vi "mainObjectivesRegistrationEtl.vi"() -> ()   [LabVIEW 2017]
uses:
  getComputerName.vi
  globalDevices.vi
  globalUtilities.vi
  <vilib>/Analysis/NI_AALBase.lvlib
panel:
  out "setting etl1 to":dbl
  out "folder name":string
  in  "redgreen":bool=TRUE
  out "Intensity Graph":u16[][](graph)
  out "XY Graph 6":cluster{"X":dbl, "Y":dbl}[](graph)
  out "XY Graph 5":cluster{"X":dbl, "Y":dbl}[](graph)
  out "XY Graph 4":cluster{"X":dbl, "Y":dbl}[](graph)
  out "XY Graph 3":cluster{"X":dbl, "Y":dbl}[](graph)
  out "XY Graph 2":cluster{"X":dbl, "Y":dbl}[](graph)
  out "XY Graph":cluster{"X":dbl, "Y":dbl}[](graph)
  out "curr etl0 pos (index)":i32
  out "dpt0[dpt1]":dbl[](array[numeric])=[-1.3290463804486958, -1.2316305979268645, -1.1212630461318092, -1.0138414017259925, -0.9077086052642437, -0.7879824961067727, -0.6552620830414349, -0.5431711241489464, -0.4247559983519593, -0.3094500332450975, -0.18905192370600912, -0.06093037048920009, 0.06463589071459266, 0.2196498896905996, 0.3584540083954262, 0.4919160251092355, 0.6311778325996011, 0.7706641387872266, 0.9159712492967972, 1.0737300085708255, 1.2329966463874322]
  in  "etl1 Q-1":i32=20
  out "N^2 +M galvo":i32
  out "curr. etl1 pos (index)":i32
  out "curr. galvo pos (index)":i32
  out "opendisplayvolume":bool=TRUE
  in  "frames per second":dbl=2.0
  in  "etl0 P-1":i32=40
  in  "galvo N-1":i32=3
  # "REGISTRATION BETWEEN GALVO AND CAMERA"
  # "To produce the Red-Green transformation, after running this VI with redgreen=true, use subvi/subvi-gmmreg/gmmregRegisterRedAndGreen."
  # "Acquisition parameters"
  # "# of etl \npositions to scan"
  # "40 20 for normal operation"
  # "sqrt# of galvo positions in grid\n(without symmetry breaking)"
  # "To set the extent of the galvo scan, use globalDevices.vi."
  # "0. No iris closed after tunable lens, lenses released, laser on, camera released."
  # "1. After the ETL scan ends, the Display Volume vi will open. Select a rectangle to locate the\n    two-photon spot.\n2. After the galvo scan ends, the Display VI will open again. Select a point where you want to shine\n    light, to test the registration."
  # "Always check that the [dpt1] values are reasonable. -->\nIf not, rerun the fits and correct, using basic/test/gaussianFitTestWithData"
  # "When this button is on, open the VI (if it hasn't opened yet by itself)\nsubvi/subvi-acquisitionUtilities/acquisitionDisplayVolume.vi"
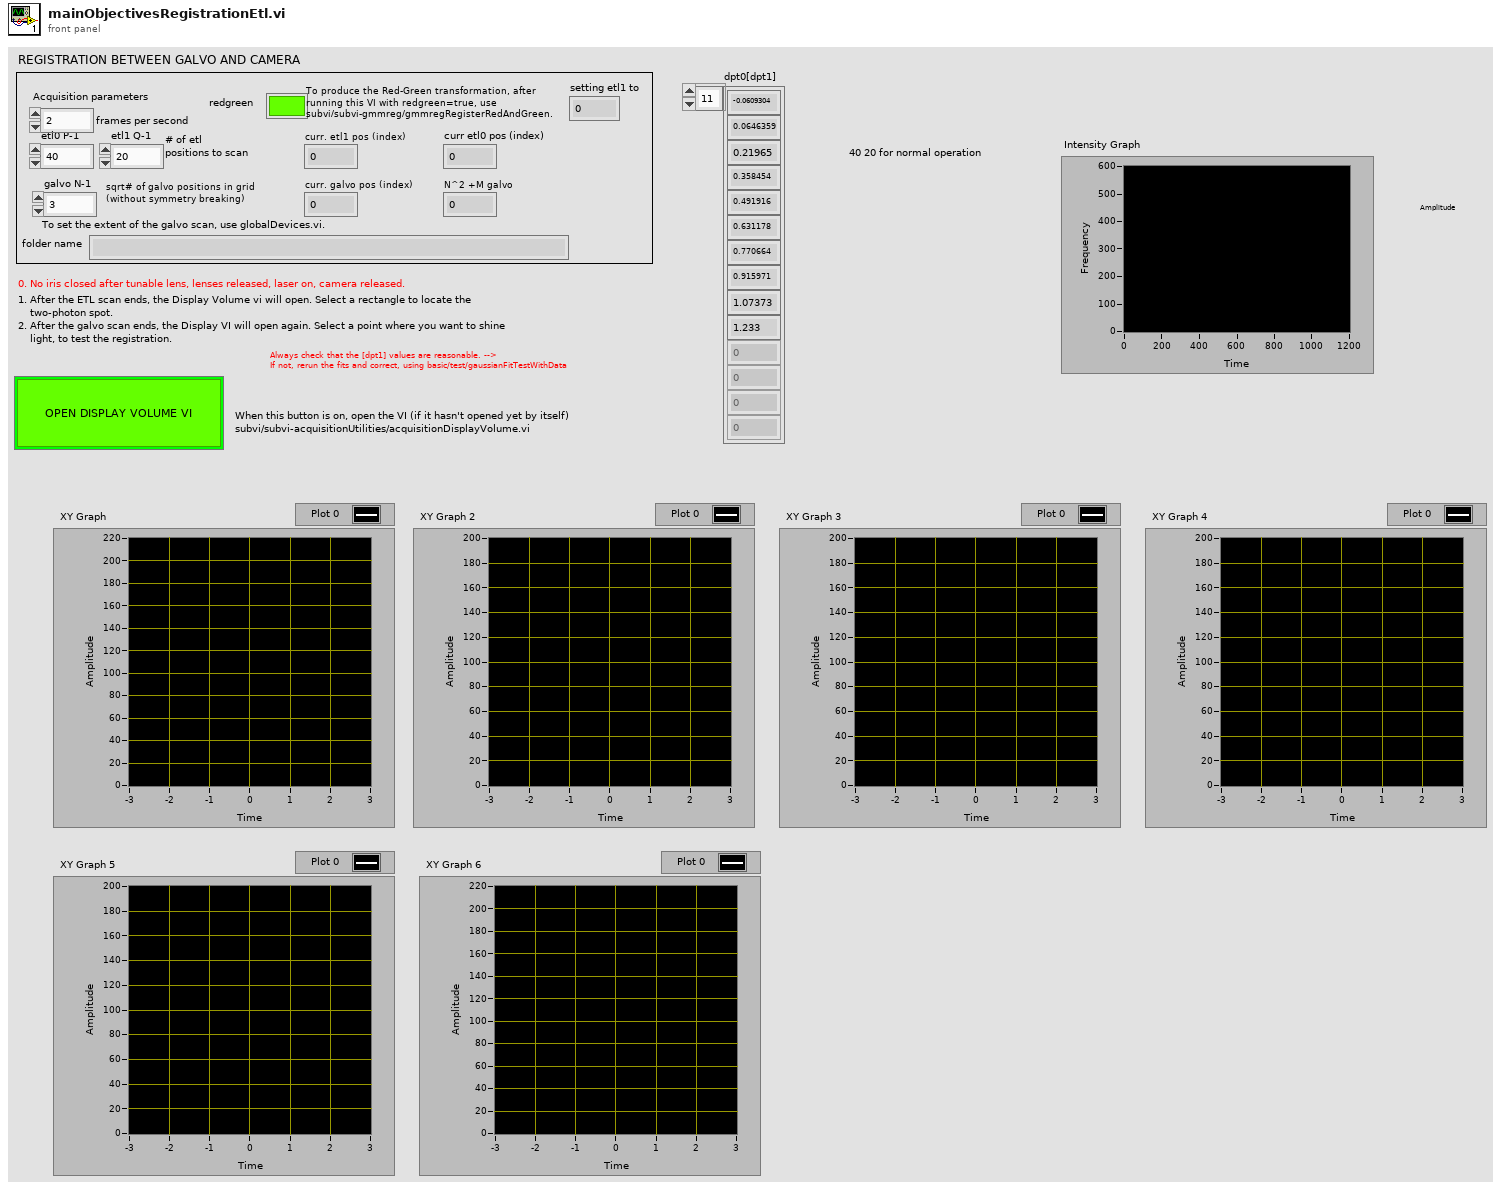
[diagram p1: front panel]
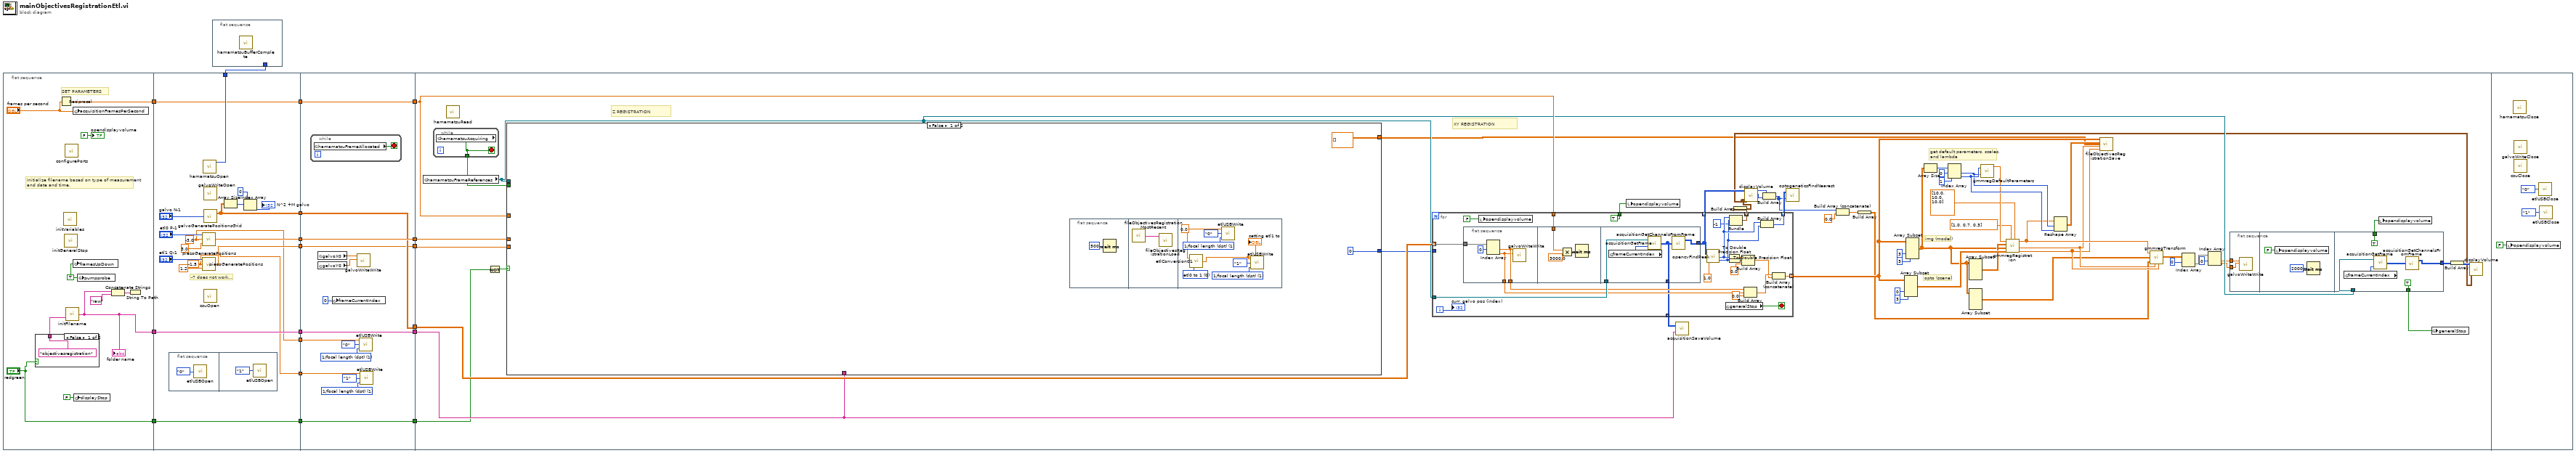
[diagram p0: block diagram]
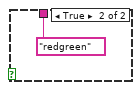
[diagram p2: hidden frame]
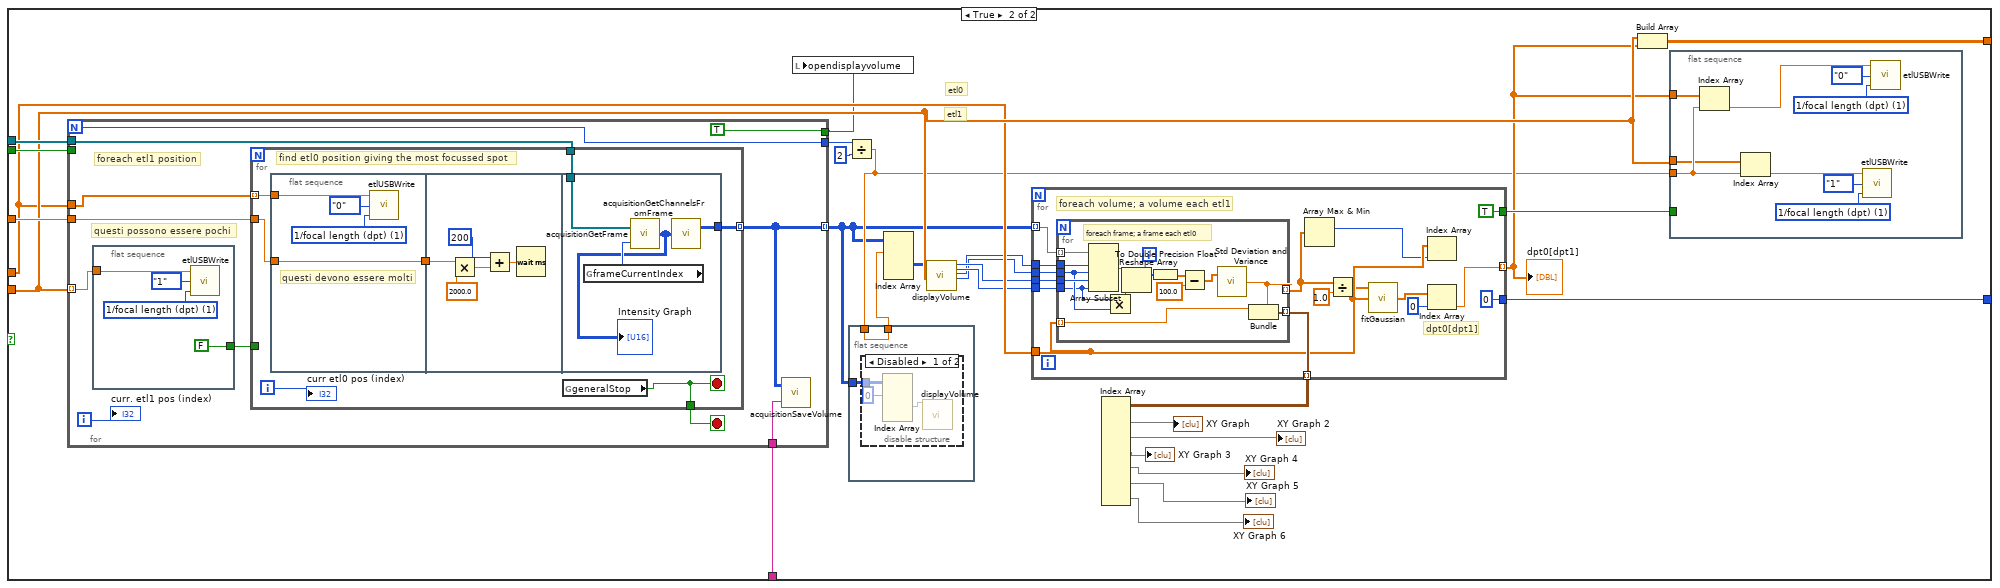
[diagram p3: hidden frame]
diagram:
  n1 = flat-sequence {
    tunnel: [w25] -> w16
    tunnel: [w22] -> w12
    tunnel: ["redgreen"] -> w7
    tunnel: [w46] -> w18
    tunnel: [w37] -> w17
    tunnel: w16 -> [w43]
    tunnel: [w43] -> w15
    tunnel: [w42] -> w14
    tunnel: [w38] -> w13
    tunnel: w12 -> [w38]
    tunnel: [w34] -> w11
    tunnel: [w32] -> w10
    tunnel: [w33] -> w9
    tunnel: [w31] -> w8
    tunnel: w7 -> [w31]
    tunnel: w17 -> [w64]
    tunnel: [w64] -> w6
    tunnel: [w63] -> w5
    tunnel: w15 -> [w63]
    tunnel: [w62] -> w4
    tunnel: w14 -> [w62]
    tunnel: [w61] -> w3
    tunnel: w13 -> [w61]
    tunnel: w11 -> [w60]
    tunnel: [w60] -> w2
    tunnel: w10 -> [w54]
    tunnel: w9 -> [w53]
    tunnel: [w50] -> w1
    tunnel: w8 -> [w50]
    tunnel: w6 -> [w69]
    tunnel: w5 -> [w117]
    tunnel: w4 -> [w119]
    tunnel: w3 -> [w68]
    tunnel: w2 -> [w70]
    tunnel: w1 -> [w67]
    frame #0 {
      w23 = TRUE ("pumpprobe")
      # "SET PARAMETERS"
      # "Initialize filename based on type of measurement\nand date and time."
      n2 = case shown="False" "redgreen" {
        tunnel: ["objectivesregistration" ("Experiment type") "redgreen" ("Experiment type")] -> w21
        frame False {
        }
        frame True {
        }
      }
      n3 = Reciprocal(x="frames per second") -> (1/x=w25:dbl)
      n4 = call "initVariables.vi"() -> ()  [unwired: 12 in]
      n5 = call "initGeneralStop.vi"() -> ()  [unwired: 1 in]
      n6 = call "configurePorts.vi"() -> ()  [unwired: 12 in]
      n7 = call "initFilename.vi"("Experiment type"=w21) -> ("folder name"=w22:string)  [unwired: 1 in]
      "folder name" <- w22
      n8 = global write "globalUtilities.vi" "framesUpDown"(w23) -> ()
      n9 = global write "globalUtilities.vi" "acquisitionFramesPerSecond"("frames per second") -> ()
      n10 = global write "globalUtilities.vi" "displayStop"(FALSE ("displayStop")) -> ()
      n11 = global write "globalUtilities.vi" "pumpprobe"(w23) -> ()
      n12 = Concatenate Strings(w22, "raw") -> (w28:string)
      n13 = String To Path(string=w28) -> ()  [unwired: 1 out]
      "opendisplayvolume" <- FALSE ("OPEN DISPLAY VOLUME")
    }
    frame #1 {
      w33 = -1.5 ("z0")
      w32 = -3.0 ("z0")
      # "-7 does not work..."
      n14 = flat-sequence {
        frame #0 {
          n15 = call "etlUSBOpen.vi"("lens"=enum16{"0", "1"}."0") -> ()  [unwired: 1 in, 1 out]
        }
        frame #1 {
          n16 = call "etlUSBOpen.vi"("lens"=enum16{"0", "1"}."1") -> ()  [unwired: 1 in, 1 out]
        }
      }
      n17 = call "piezoGeneratePositions.vi"("zf"=1.2, "z0"=w33, "M"="etl1 Q-1") -> ("positions (z)"=w34:dbl[])
      n18 = call "piezoGeneratePositions.vi"("zf"=3.0, "z0"=w32, "M"="etl0 P-1") -> ("positions (z)"=w37:dbl[])
      n19 = call "hamamatsuOpen.vi"() -> ("Handle out"=w46:u32)  [unwired: 3 out]
      n20 = call "galvoWriteOpen.vi"() -> ()  [unwired: 12 in]
      n21 = call "galvoGeneratePositionsGrid.vi"("N-1"="galvo N-1") -> ("grid"=w42:dbl[][])  [unwired: 1 out]
      n22 = call "csuOpen.vi"() -> ()  [unwired: 14 in, 2 out]
      n23 = Array Size(array=w42) -> (size(s)=w41:i32[])
      n24 = Index Array(array=w41, index=0) -> (element=→"N^2 +M galvo":i32)
    }
    frame #2 {
      w55 = u16 1 items=["position (um)", "1/focal length (dpt)"] ("mode")
      w58 = u16 1 items=["position (um)", "1/focal length (dpt)"] ("mode")
      n25 = while {
        stop <- w65 stop-if-true
        n26 = global read "globalDevices.vi" "hamamatsuFrameAllocated"() -> (w65:bool)
      }
      n27 = global read "globalDevices.vi" "galvoX0"() -> (w52:dbl)
      n28 = global read "globalDevices.vi" "galvoY0"() -> (w51:dbl)
      n29 = global write "globalUtilities.vi" "frameCurrentIndex"(0 ("frameCurrentIndex")) -> ()
      n30 = call "galvoWriteWrite.vi"("X"=w52, "Y"=w51) -> ()  [unwired: 4 in]
      n31 = call "etlUSBWrite.vi"("mode"=w55, "lens"=enum16{"0", "1"}."0", "input"=w54) -> ()  [unwired: 1 in]
      n32 = call "etlUSBWrite.vi"("mode"=w58, "lens"=enum16{"0", "1"}."1", "input"=w53) -> ()  [unwired: 1 in]
    }
    frame #3 {
      # "XY REGISTRATION"
      # "Z REGISTRATION"
      # "get default parameters, scales,\nand lambda"
      # "img (model)"
      # "opto (scene)"
      n33 = global read "globalDevices.vi" "hamamatsuFrameReferences"() -> (w96:refnum<data-value>[])
      n34 = while {
        tunnel: [w283] -> w118
        stop <- w283 stop-if-true
        n35 = global read "globalUtilities.vi" "hamamatsuAcquiring"() -> (w283:bool)
      }
      n36 = call "hamamatsuRead.vi"() -> ()  [unwired: 12 in]
      n37 = Not(x=w67) -> (.not. x?=w66:bool)
      n38 = case shown="False" w66 {
        tunnel: w118 -> [_ w158]
        tunnel: w117 -> [_ w157]
        tunnel: w96 -> [_ w156]
        tunnel: [0 w155] -> w72
        tunnel: [dbl[][] [] w154] -> w71
        tunnel: w70 -> [_ w153]
        tunnel: w69 -> [_ w150]
        tunnel: w68 -> [_ w148]
        frame False {
          n39 = flat-sequence {
            frame #0 {
              n40 = Wait (ms)(milliseconds to wait=u32 500) -> ()  [unwired: 1 out]
            }
            frame #1 {
              n41 = call "fileObjectivesRegistrationMostRecent.vi"() -> ("f"=w123:string)  [unwired: 1 in]
              n42 = call "fileObjectivesRegistrationLoad.vi"("objectiveRegistrationFilePath"=w123) -> ()  [unwired: 3 in, 6 out]
            }
            frame #2 {
              w125 = u16 0 items=["etl0 to 1", "etl1 to 0"] ("mode")
              w126 = 0.0 ("input")
              w130 = u16 1 items=["position (um)", "1/focal length (dpt)"] ("mode")
              w127 = u16 1 items=["position (um)", "1/focal length (dpt)"] ("mode")
              n43 = call "etlConversion01.vi"("mode"=w125, "in"=w126) -> ("out"=w124:dbl)
              "setting etl1 to" <- w124
              n44 = call "etlUSBWrite.vi"("mode"=w130, "lens"=enum16{"0", "1"}."0", "input"=w126) -> ()  [unwired: 1 in]
              n45 = call "etlUSBWrite.vi"("mode"=w127, "lens"=enum16{"0", "1"}."1", "input"=w124) -> ()  [unwired: 1 in]
            }
          }
        }
        frame True {
          # "etl0"
          # "etl1"
          n46 = for {
            N -> [w200]
            tunnel: w156 -> [w201]
            tunnel: w157 -> [w202]
            tunnel: [TRUE] -> w147
            tunnel: w158 -> [_]
            tunnel: [w194] -> w131 mode=indexing
            tunnel: [w200] -> w146
            tunnel: w153 -> [w199] mode=indexing
            tunnel: w150 -> [w198]
            tunnel: w148 -> [w195]
            i -> [w203]
            stop <- w196 stop-if-true
            # "foreach etl1 position"
            # "questi possono essere pochi"
            n47 = flat-sequence {
              tunnel: w199 -> [w228]
              tunnel: [FALSE] -> w197
              frame #0 {
                w226 = u16 1 items=["position (um)", "1/focal length (dpt)"] ("mode")
                n48 = call "etlUSBWrite.vi"("mode"=w226, "lens"=enum16{"0", "1"}."1", "input"=w228) -> ()  [unwired: 1 in]
              }
            }
            n49 = for {
              tunnel: w198 -> [w211] mode=indexing
              tunnel: w202 -> [w209]
              tunnel: w201 -> [w208]
              tunnel: [w207] -> w194 mode=indexing
              tunnel: w197 -> [_]
              tunnel: [w205] -> w196
              i -> [w206]
              stop <- w205 stop-if-true
              # "find etl0 position giving the most focussed spot"
              n50 = flat-sequence {
                tunnel: w211 -> [w213]
                tunnel: [w212] -> w210
                tunnel: w209 -> [w212]
                tunnel: w210 -> [w218]
                tunnel: w208 -> [w223]
                tunnel: [w222] -> w207
                frame #0 {
                  w215 = u16 1 items=["position (um)", "1/focal length (dpt)"] ("mode")
                  # "questi devono essere molti"
                  n51 = call "etlUSBWrite.vi"("mode"=w215, "lens"=enum16{"0", "1"}."0", "input"=w213) -> ()  [unwired: 1 in]
                }
                frame #1 {
                  n52 = Multiply(x=w218, y=2000.0) -> (x*y=w216:dbl)
                  n53 = Add(x=200, y=w216) -> (x+y=w220:dbl)
                  n54 = Wait (ms)(milliseconds to wait=w220) -> ()  [unwired: 1 out]
                }
                frame #2 {
                  n55 = global read "globalUtilities.vi" "frameCurrentIndex"() -> (w224:i32)
                  n56 = call "acquisitionGetFrame.vi"("index"=w224, "hamamatsuFrameReferences"=w223) -> ("frameOut"=w221:u16[][])
                  "Intensity Graph" <- w221
                  n57 = call "acquisitionGetChannelsFromFrame.vi"("frameIn"=w221) -> ("Red"=w222:u16[][])  [unwired: 1 out]
                }
              }
              n58 = global read "globalUtilities.vi" "generalStop"() -> (w205:bool)
              "curr etl0 pos (index)" <- w206
            }
            n59 = call "acquisitionSaveVolume.vi"("folder"=w195, "volume"=w194) -> ()  [unwired: 1 in]
            "curr. etl1 pos (index)" <- w203
          }
          n60 = local write "opendisplayvolume"(w147) -> ()
          n61 = Divide(x=w146, y=2) -> (x/y=w149:dbl)
          n62 = flat-sequence {
            tunnel: w149 -> [w160]
            tunnel: [w160] -> w132
            tunnel: w131 -> [w159]
            frame #0 {
              n63 = disable-structure shown="Disabled" {
                disable-tunnel: w159 -> [w163 _]
                frame Disabled {
                  n64 = Index Array(array=w163, index (dim 0)=0 ("index (vol)")) -> (element=w161:u16[][][])  [unwired: 3 in]
                  n65 = call "displayVolume.vi"("frames"=w161) -> ()  [unwired: 13 in, 6 out]
                }
                frame Enabled {
                }
              }
            }
          }
          n66 = Index Array(array=w131, index (dim 0)=w132) -> (element=w144:u16[][][])  [unwired: 3 in]
          n67 = call "displayVolume.vi"("frames"=w144, "z"=w153) -> ("X0out"=w143:i32, "deltaXout"=w142:i32, "Y0out"=w141:i32, "deltaYout"=w140:i32)  [unwired: 12 in, 2 out]
          n68 = for {
            tunnel: w131 -> [w174] mode=indexing
            tunnel: w143 -> [w179]
            tunnel: w142 -> [w178]
            tunnel: w141 -> [w177]
            tunnel: w140 -> [w176]
            tunnel: [w167] -> w151 mode=indexing
            tunnel: [0] -> w155
            tunnel: w150 -> [w169]
            tunnel: [TRUE] -> w152
            tunnel: [w170] -> w139 mode=indexing
            # "dpt0[dpt1]"
            # "foreach volume; a volume each etl1"
            n69 = for {
              tunnel: w174 -> [w193] mode=indexing
              tunnel: w179 -> [w192]
              tunnel: w178 -> [w188]
              tunnel: w177 -> [w191]
              tunnel: w176 -> [w189]
              tunnel: [w180] -> w166 mode=indexing
              tunnel: w169 -> [w186] mode=indexing
              tunnel: [w185] -> w170 mode=indexing
              # "foreach frame; a frame each etl0"
              n70 = Array Subset(array=w193, index (row)=w191, length (row)=w189, index (col)=w192, length (col)=w188) -> (w190:u16[][])
              n71 = Multiply(x=w188, y=w189) -> (x*y=w187:i32)
              n72 = Reshape Array(w190, w187) -> (w184:u16[])
              n73 = To Double Precision Float(number=w184) -> (double precision float=w183:dbl[])
              n74 = Subtract(x=w183, y=100.0) -> (x-y=w182:dbl[])
              n75 = call <vilib>:"Std Deviation and Variance.vi"("X"=w182) -> ("standard deviation"=w180:dbl)  [unwired: 1 in, 2 out]
              n76 = Bundle(w186, "standard deviation"=w180) -> (w185:cluster{dbl, "standard deviation":dbl})  [unwired: 1 in]
            }
            n77 = Array Max & Min(array=w166) -> (max index (indices)=w168:i32)  [unwired: 3 out]
            n78 = Divide(x=w166, y=1.0) -> (x/y=w165:dbl[])
            n79 = call "fitGaussian.vi"("X"=w169, "Y"=w165) -> ("x0,sigma,bg,amplitude"=w172:dbl[])  [unwired: 1 in]
            n80 = Index Array(array=w169, index=w168) -> ()  [unwired: 1 out]
            n81 = Index Array(array=w172, index=0) -> (element=w167:dbl)
          }
          "dpt0[dpt1]" <- w151
          n82 = Index Array(array=w139) -> (element #1=→"XY Graph":cluster{dbl, "standard deviation":dbl}[], element #2=→"XY Graph 2":cluster{dbl, "standard deviation":dbl}[], element #3=→"XY Graph 3":cluster{dbl, "standard deviation":dbl}[], element #4=→"XY Graph 4":cluster{dbl, "standard deviation":dbl}[], element #5=→"XY Graph 5":cluster{dbl, "standard deviation":dbl}[], element #6=→"XY Graph 6":cluster{dbl, "standard deviation":dbl}[])  [unwired: 12 in]
          n83 = Build Array(w153, w151) -> (w154:dbl[][])
          n84 = flat-sequence {
            tunnel: w151 -> [w232]
            tunnel: w149 -> [w231]
            tunnel: w153 -> [w229]
            tunnel: w152 -> [_]
            frame #0 {
              w235 = u16 1 items=["position (um)", "1/focal length (dpt)"] ("mode")
              w236 = u16 1 items=["position (um)", "1/focal length (dpt)"] ("mode")
              n85 = Index Array(array=w232, index=w231) -> (element=w230:dbl)
              n86 = Index Array(array=w229, index=w231) -> (element=w233:dbl)
              n87 = call "etlUSBWrite.vi"("mode"=w235, "lens"=enum16{"0", "1"}."1", "input"=w233) -> ()  [unwired: 1 in]
              n88 = call "etlUSBWrite.vi"("mode"=w236, "lens"=enum16{"0", "1"}."0", "input"=w230) -> ()  [unwired: 1 in]
            }
          }
        }
      }
      n89 = for {
        tunnel: w119 -> [w271] mode=indexing
        tunnel: w117 -> [w270]
        tunnel: w96 -> [w269]
        tunnel: [w266] -> w116 mode=indexing
        tunnel: [w265] -> w75 mode=indexing
        tunnel: [w257] -> w102 mode=indexing
        tunnel: [w255] -> w99 mode=indexing
        tunnel: [TRUE ("OPEN DISPLAY VOLUME")] -> w77
        tunnel: [w249] -> w73 mode=indexing
        tunnel: w72 -> [_]
        i -> [w267]
        stop <- w248 stop-if-true
        n90 = flat-sequence {
          tunnel: w271 -> [w275]
          tunnel: [w273] -> w261
          tunnel: [w272] -> w260
          tunnel: w270 -> [w277]
          tunnel: w269 -> [w281]
          tunnel: [w280] -> w266
          tunnel: [w279] -> w249
          frame #0 {
            n91 = Index Array(array=w275, index #1=0 ("index")) -> (element #1=w273:dbl, element #2=w272:dbl)  [unwired: 1 in]
            n92 = call "galvoWriteWrite.vi"("X"=w273, "Y"=w272) -> ()  [unwired: 4 in]
          }
          frame #1 {
            n93 = Multiply(x=w277, y=3000.0) -> (x*y=w276:dbl)
            n94 = Wait (ms)(milliseconds to wait=w276) -> ()  [unwired: 1 out]
          }
          frame #2 {
            n95 = global read "globalUtilities.vi" "frameCurrentIndex"() -> (w282:i32)
            n96 = call "acquisitionGetFrame.vi"("index"=w282, "hamamatsuFrameReferences"=w281) -> ("frameOut"=w279:u16[][])
            n97 = call "acquisitionGetChannelsFromFrame.vi"("frameIn"=w279) -> ("Red"=w280:u16[][])  [unwired: 1 out]
          }
        }
        n98 = local write "opendisplayvolume"(FALSE ("OPEN DISPLAY VOLUME")) -> ()
        n99 = call "opencvFindPeak.vi"("blur"=1.0, "Image (2D)"=w266) -> ("maxLocY"=w254:i32, "maxLocX"=w256:i32)
        n100 = global read "globalUtilities.vi" "generalStop"() -> (w248:bool)
        n101 = To Double Precision Float(number=w256) -> (double precision float=w263:dbl)
        n102 = To Double Precision Float(number=w254) -> (double precision float=w262:dbl)
        n103 = Bundle("maxLocX"=w256, "maxLocY"=w254, -1) -> (w265:cluster{"maxLocX":i32, "maxLocY":i32, i32})  [unwired: 1 in]
        n104 = Build Array(w263, w262, 0.0 ("element")) -> (w253:dbl[])
        n105 = Build Array(w261, w260, 0.0 ("element")) -> (w258:dbl[])
        n106 = Build Array(w256, w254) -> (w255:i32[])
        n107 = Build Array (concatenate)(w258, w253) -> (w257:dbl[])
        "curr. galvo pos (index)" <- w267
      }
      n108 = local write "opendisplayvolume"(w77) -> ()
      n109 = call "acquisitionSaveVolume.vi"("folder"=w68, "volume"=w73) -> ()  [unwired: 1 in]
      n110 = Build Array(w75) -> (w74:cluster{"maxLocX":i32, "maxLocY":i32, i32}[][])
      n111 = call "displayVolume.vi"("frames"=w116, "overlay (z:-1 all planes)"=w74) -> ("X0out"=w115:i32, "Y0out"=w114:i32)  [unwired: 12 in, 4 out]
      n112 = Build Array(w115, w114) -> (w81:i32[])
      n113 = call "optogeneticsFindNearest.vi"("point"=w81, "points"=w99) -> ()  [unwired: 1 out]
      n114 = Build Array (concatenate)(w81, 0.0) -> (w79:dbl[])
      n115 = Build Array(w79) -> (w78:dbl[][])
      n116 = Array Subset(array=w102, index (col)=0 ("index"), length (col)=3 ("length")) -> (w91:dbl[][])  [unwired: 2 in]
      n117 = Array Subset(array=w102, index (col)=3 ("index"), length (col)=3 ("length")) -> (w89:dbl[][])  [unwired: 2 in]
      n118 = Array Size(array=w89) -> (size(s)=w109:i32[])
      n119 = Index Array(array=w109, index #1=0 ("index"), index #2=1 ("index")) -> (element #1=w111:i32, element #2=w112:i32)
      n120 = Array Subset(array=w89) -> (w88:dbl[][])  [unwired: 4 in]
      n121 = Array Subset(array=w89) -> (w90:dbl[][])  [unwired: 4 in]
      n122 = call "gmmregDefaultParameters.vi"("D (3)"=w112, "nctrlPts"=w111) -> ("param0"=w110:dbl[])  [unwired: 3 out]
      n123 = call "gmmregRegistration.vi"("lambda"=dbl[] [10.0, 10.0, 10.0], "scale"=dbl[] [1.0, 0.7, 0.3], "scene"=w91, "model"=w89, "ctrlPoints"=w90, "param0"=w110) -> ("denormParams out"=w92:dbl[], "normParams out"=w100:dbl[], "param0 out"=w101:dbl[])  [unwired: 2 in, 1 out]
      n124 = Reshape Array(w101, w111, w112) -> (w113:dbl[][])
      n125 = call "fileObjectivesRegistrationSave.vi"("xyz(opto)xyz(img)"=w102, "param"=w113, "normParam"=w100, "denormParam"=w92, "z(opto)z(img)"=w71) -> ()  [unwired: 1 in]
      n126 = call "gmmregTransform.vi"("param0"=w101, "ctrlPts"=w88, "pts"=w78, "normParams"=w100, "denormParams"=w92) -> ("out"=w98:dbl[][])  [unwired: 4 in]
      n127 = Index Array(array=w98, index (row)=0) -> (element=w87:dbl[])  [unwired: 1 in]
      n128 = Index Array(array=w87, index #1=0 ("index")) -> (element #1=w85:dbl, element #2=w84:dbl)  [unwired: 1 in]
      n129 = flat-sequence {
        tunnel: w85 -> [w239]
        tunnel: w84 -> [w238]
        tunnel: w96 -> [w246]
        tunnel: [w242] -> w95
        tunnel: [TRUE] -> w93
        tunnel: [TRUE ("opendisplayvolume")] -> w76
        frame #0 {
          n130 = call "galvoWriteWrite.vi"("X"=w239, "Y"=w238) -> ()  [unwired: 4 in]
        }
        frame #1 {
          n131 = local write "opendisplayvolume"(FALSE ("opendisplayvolume")) -> ()
          n132 = Wait (ms)(milliseconds to wait=u32 2000) -> ()  [unwired: 1 out]
        }
        frame #2 {
          n133 = global read "globalUtilities.vi" "frameCurrentIndex"() -> (w247:i32)
          n134 = call "acquisitionGetFrame.vi"("index"=w247, "hamamatsuFrameReferences"=w246) -> ("frameOut"=w243:u16[][])
          n135 = call "acquisitionGetChannelsFromFrame.vi"("frameIn"=w243) -> ("Red"=w242:u16[][])  [unwired: 1 out]
        }
      }
      n136 = local write "opendisplayvolume"(w76) -> ()
      n137 = global write "globalUtilities.vi" "generalStop"(w93) -> ()
      n138 = Build Array(w95) -> (w94:u16[][][])
      n139 = call "displayVolume.vi"("frames"=w94, "overlay (z:-1 all planes)"=w74) -> ()  [unwired: 12 in, 6 out]
    }
    frame #4 {
      n140 = local write "opendisplayvolume"(FALSE ("opendisplayvolume")) -> ()
      n141 = call "hamamatsuClose.vi"() -> ()  [unwired: 1 out]
      n142 = call "galvoWriteClose.vi"() -> ()  [unwired: 12 in]
      n143 = call "csuClose.vi"() -> ()  [unwired: 12 in]
      n144 = call "etlUSBClose.vi"("lens"=enum16{"0", "1"}."0") -> ()  [unwired: 1 in]
      n145 = call "etlUSBClose.vi"("lens"=enum16{"0", "1"}."1") -> ()  [unwired: 1 in]
    }
  }
  n146 = flat-sequence {
    tunnel: w18 -> [_]
    frame #0 {
      n147 = call "hamamatsuBufferComplete.vi"() -> ()  [unwired: 12 in]
    }
  }
